vi "KVMap-To String.vi"(11 "Cluster":cluster{string[], string[]}) -> (3 "value":string)   [LabVIEW 2014]
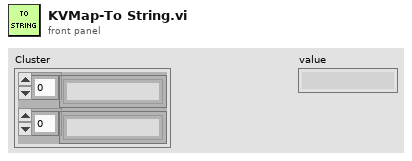
[diagram p1: front panel]
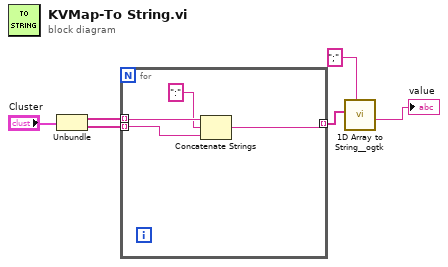
[diagram p0: block diagram]
diagram:
  n1 = Unbundle("Cluster") -> (w5:string[], w4:string[])
  n2 = for {
    tunnel: w5 -> [w10] mode=indexing
    tunnel: w4 -> [w9] mode=indexing
    tunnel: [w7] -> w3 mode=indexing
    n3 = Concatenate Strings(w10, ":" ("string"), w9) -> (w7:string)
  }
  n4 = call <userlib>:"1D Array to String__ogtk.vi"("delimiter (Tab)"=";", "Array of Strings"=w3) -> ("delimited string"=→"value":string)  [unwired: 9 in]
